vi "Equip-Get AI Channels.vi"(7 "Inputs":T1[](array[typedef]) items=["--unused--", "Probe Mic Right", "Probe Mic Left", "Cal Mic", "ABR", "CAP Right", "CAP Left", "Startle piezo", "Temperature", "Heart rate", "Accelerometer", "Startle piezo 2"], 11 "error in (no error)":errorcluster) -> (8 "AI Channels":i32[](array[numeric]), 15 "error out":errorcluster)   [LabVIEW 2020]
uses:
  Type Defs/Input sources.ctl
  <vilib>/Utility/config.llb/Read Key (I32).vi
  <vilib>/Utility/config.llb/NI_LVConfig.lvlib
panel:
  in  "Input sources":T1 items=["--unused--", "Probe Mic Right", "Probe Mic Left", "Cal Mic", "ABR", "CAP Right", "CAP Left", "Startle piezo", "Temperature", "Heart rate", "Accelerometer", "Startle piezo 2"]
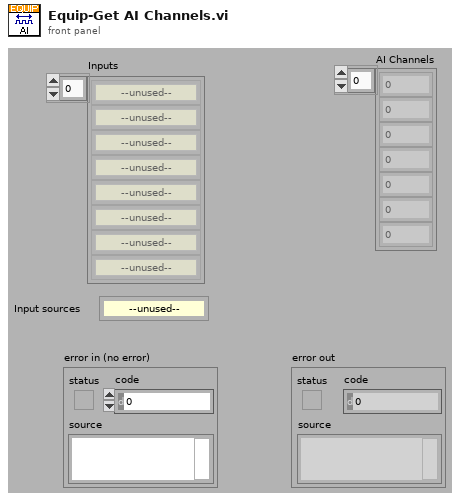
[diagram p1: front panel]
types:
  T1 = typedef "Input sources.ctl" = u16
  T2 = typedef "NI_LVConfig.lvlib/Config Data RefNum.ctl" = refnum<k1>
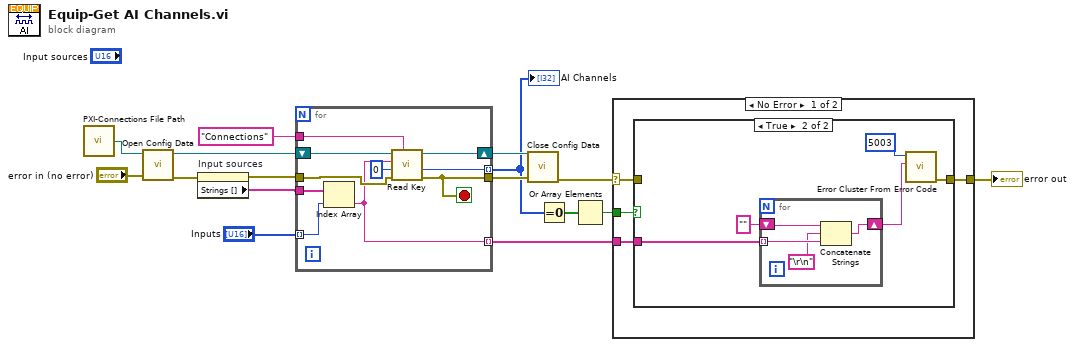
[diagram p0: block diagram]
diagram:
  n1 = call "PXI-Connections File Path.vi"() -> ("Path"=w1:path)  [unwired: 1 in]
  n2 = call <vilib>:"Open Config Data.vi"("error in (no error)"="error in (no error)", "configuration file path"=w1) -> ("error out"=w5:errorcluster, "refnum"=w4:T2)  [unwired: 7 in, 1 out]
  n3 = property on="Input sources" class="Ring (strict)"(error in=w5) -> (error out=w6:errorcluster, "Strings []"=w7:string[])  [unwired: 1 in, 1 out]
  n4 = for {
    tunnel: "Inputs" -> [w18] mode=indexing
    tunnel: w7 -> [w26]
    tunnel: [w22] -> w12 mode=indexing
    tunnel: "Connections" ("section") -> [w20]
    tunnel: w6 -> [w25]
    tunnel: [w19] -> w14
    tunnel: [w17] -> w2 mode=indexing
    shift-right: [w21] -> w13
    shift-left: w4 -> [w24]
    stop <- w19 stop-if-true
    n5 = Index Array(array=w26, index=w18) -> (element=w17:string)
    n6 = call-poly <vilib>:"Read Key.vi"("section"=w20, "error in (no error)"=w25, "default value"=0, "key"=w17, "refnum"=w24) -> ("error out"=w19:errorcluster, "value"=w22:i32, "refnum out"=w21:T2)  [unwired: 3 in, 1 out]
  }
  "AI Channels" <- w12
  n7 = call <vilib>:"Close Config Data.vi"("error in (no error)"=w14, "refnum"=w13) -> ("error out"=w8:errorcluster)  [unwired: 8 in, 1 out]
  n8 = Equal To 0?(x=w12) -> (x = 0?=w11:bool[])
  n9 = Or Array Elements(Boolean array=w11) -> (logical OR=w10:bool)
  n10 = case shown="No Error" w8 {
    selector: w8 -> [w28 w41]
    tunnel: w10 -> [w30 _]
    tunnel: [w29 w41] -> w9
    tunnel: w2 -> [w27 _]
    frame No Error {
      n11 = case shown="True" w30 {
        tunnel: w28 -> [w31 _]
        tunnel: [w31 w36] -> w29
        tunnel: w27 -> [_ w34]
        frame False {
        }
        frame True {
          n12 = for {
            tunnel: w34 -> [w39] mode=indexing
            shift-right: [w40] -> w33
            shift-left: "" -> [w37]
            n13 = Concatenate Strings(w37, "\r\n", w39) -> (w40:string)
          }
          n14 = call <vilib>:"Error Cluster From Error Code.vi"("error message (\"\")"=w33, "error code (0)"=5003) -> ("error out"=w36:errorcluster)  [unwired: 7 in]
        }
      }
    }
    frame Error {
    }
  }
  "error out" <- w9
